vi "log analysis_gps.vi"() -> ()   [LabVIEW 2018] (continued)
283169.300,02000000,471d,15824;INS_ALIGNMENT_COMPLETE,INS_RTKFIXED,37.37108798474,126.72336907996,8.2218,22.3000,0.0121,0.0069,-0.0018,-0.383839466,-0.586517581,287.881593098,0.2239,0.1710,0.2714,0.0357,0.0355,0.0323,0.0788,0.0798,5.0127,0f000005,0*36e8c713\n\tsystem status\tnormal 2 28.000000 0 0\trobot status\t224.455343\t106.296732\t8.221800\t-0.383839\t-0.586518\t162.118407\t0.000000\t0.000000\n\t\n15:39:11.8\tlog_raw\tgps_raw\t#INSPVAXA,USB3,0,47.5,FINESTEERING,2107,283169.800,02000000,471d,15824;INS_ALIGNMENT_COMPLETE,INS_RTKFIXED,37.37108797168,126.72336907326,8.2216,22.3000,0.0108,0.0060,-0.0021,-0.382641749,-0.586060307,287.885088335,0.2239,0.1710,0.2714,0.0357,0.0355,0.0323,0.0788,0.0798,5.0127,0f000005,0*d441264a\n\tsystem status\tnormal 2 28.000000 0 0\trobot status\t224.454749\t106.295283\t8.221600\t-0.382642\t-0.586060\t162.114912\t0.000000\t0.000000\n\t\n15:39:12.3\tlog_raw\tgps_raw\t#INSPVAXA,USB3,0,49.5,FINESTEERING,2107,283170.300,02000000,471d,15824;INS_ALIGNMENT_COMPLETE,INS_RTKFIXED,37.37108796269,126.72336906818,8.2217,22.3000,0.0104,0.0055,-0.0014,-0.383475872,-0.583542182,287.889042259,0.2231,0.1689,0.2708,0.0348,0.0347,0.0316,0.0786,0.0797,5.0142,0f000005,0*32689bb7\n\tsystem status\tnormal 2 28.000000 0 0\trobot status\t224.454300\t106.294285\t8.221700\t-0.383476\t-0.583542\t162.110958\t0.000000\t0.000000\n\t\n15:39:12.8\tlog_raw\tgps_raw\t#INSPVAXA,USB3,0,49.5,FINESTEERING,2107,283170.800,02000000,471d,15824;INS_ALIGNMENT_COMPLETE,INS_RTKFIXED,37.37108796102,126.72336906813,8.2219,22.3000,0.0104,0.0056,-0.0013,-0.382678847,-0.583610963,287.888842190,0.2231,0.1689,0.2708,0.0348,0.0347,0.0316,0.0786,0.0797,5.0142,0f000005,0*5e85f202\n\tsystem status\tnormal 2 28.000000 0 0\trobot status\t224.454295\t106.294100\t8.221900\t-0.382679\t-0.583611\t162.111158\t0.000000\t0.000000\n\t\n15:39:13.3\tlog_raw\tgps_raw\t#INSPVAXA,USB3,0,48.5,FINESTEERING,2107,283171.300,02000000,471d,15824;INS_ALIGNMENT_COMPLETE,INS_RTKFIXED,37.37108796031,126.72336906830,8.2221,22.3000,0.0098,0.0065,-0.0020,-0.382671205,-0.583618137,287.888068003,0.2220,0.1670,0.2703,0.0345,0.0344,0.0314,0.0786,0.0797,5.0156,0f000005,0*d6c1e6dd\n\tsystem status\tnormal 2 28.000000 0 0\trobot status\t224.454310\t106.294021\t8.222100\t-0.382671\t-0.583618\t162.111932\t0.000000\t0.000000\n\t\n15:39:13.8\tlog_raw\tgps_raw\t#INSPVAXA,USB3,0,48.5,FINESTEERING,2107,283171.800,02000000,471d,15824;INS_ALIGNMENT_COMPLETE,INS_RTKFIXED,37.37108796545,126.72336907471,8.2220,22.3000,0.0105,0.0071,-0.0022,-0.380415359,-0.582586820,287.889750442,0.2220,0.1670,0.2703,0.0345,0.0344,0.0314,0.0786,0.0797,5.0156,0f000005,0*ca9dcfb0\n\tsystem status\tnormal 2 28.000000 0 0\trobot status\t224.454878\t106.294591\t8.222000\t-0.380415\t-0.582587\t162.110250\t0.000000\t0.000000\n\t\n15:39:14.3\tlog_raw\tgps_raw\t#INSPVAXA,USB3,0,50.0,FINESTEERING,2107,283172.300,02000000,471d,15824;INS_ALIGNMENT_COMPLETE,INS_RTKFIXED,37.37108796771,126.72336907645,8.2222,22.3000,0.0108,0.0068,-0.0016,-0.379539912,-0.580787545,287.890138856,0.2209,0.1652,0.2698,0.0344,0.0343,0.0313,0.0787,0.0798,5.0170,0f000005,0*259de970\n\tsystem status\tnormal 2 28.000000 0 0\trobot status\t224.455032\t106.294842\t8.222200\t-0.379540\t-0.580788\t162.109861\t0.000000\t0.000000\n\t\n15:39:14.8\tlog_raw\tgps_raw\t#INSPVAXA,USB3,0,50.0,FINESTEERING,2107,283172.800,02000000,471d,15824;INS_ALIGNMENT_COMPLETE,INS_RTKFIXED,37.37108797403,126.72336907678,8.2227,22.3000,0.0110,0.0071,-0.0014,-0.379066228,-0.579747038,287.892022667,0.2209,0.1652,0.2698,0.0344,0.0343,0.0313,0.0787,0.0798,5.0170,0f000005,0*0ecf865b\n\tsystem status\tnormal 2 28.000000 0 0\trobot status\t224.455061\t106.295543\t8.222700\t-0.379066\t-0.579747\t162.107977\t0.000000\t0.000000\n\t\n15:39:15.3\tlog_raw\tgps_raw\t#INSPVAXA,USB3,0,51.5,FINESTEERING,2107,283173.300,02000000,471d,15824;INS_ALIGNMENT_COMPLETE,INS_RTKFIXED,37.37108801209,126.72336910611,8.2226,22.3000,0.0136,0.0085,-0.0010,-0.377696334,-0.579038466,287.894073906,0.2209,0.1652,0.2698,0.0344,0.0343,0.0313,0.0787,0.0798,5.0170,0f000005,0*92cf69d3\n\tsystem status\tnormal 2 28.000000 0 0\trobot status\t224.457659\t106.299767\t8.222600\t-0.377696\t-0.579038\t162.105926\t0.000000\t0.000000\n\t\n15:39:15.8\tlog_raw\tgps_raw\t#INSPVAXA,USB3,0,51.5,FINESTEERING,2107,283173.800,02000000,471d,15824;INS_ALIGNMENT_COMPLETE,INS_RTKFIXED,37.37108808085,126.72336916289,8.2221,22.3000,0.0168,0.0112,-0.0008,-0.373536353,-0.577127426,287.890111312,0.2209,0.1652,0.2698,0.0344,0.0343,0.0313,0.0787,0.0798,5.0170,0f000005,0*81360348\n\tsystem status\tnormal 2 28.000000 0 0\trobot status\t224.462689\t106.307399\t8.222100\t-0.373536\t-0.577127\t162.109889\t0.000000\t0.000000\n\t\n15:39:16.3\tlog_raw\tgps_raw\t#DUALANTENNAHEADINGA,USB3,0,44.0,FINESTEERING,2107,283174.300,02000000,d426,15824;INSUFFICIENT_OBS,NONE,-1.000000000,0.000000000,0.000000000,0.0,0.000000000,0.000000000,\"631T\",17,4,4,3,04,00,20,03*70a0cfeb\n\tsystem status\tnormal 2 28.000000 0 0\trobot status\t224.463323\t106.308276\t8.222100\t-0.371384\t-0.577439\t162.106720\t0.000000\t0.000000\n\t\n15:39:16.8\tlog_raw\tgps_raw\t#DUALANTENNAHEADINGA,USB3,0,44.0,FINESTEERING,2107,283174.800,02000000,d426,15824;INSUFFICIENT_OBS,NONE,-1.000000000,0.000000000,0.000000000,0.0,0.000000000,0.000000000,\"631T\",15,4,4,3,04,00,20,03*9126eb2e\n\tsystem status\tnormal 2 28.000000 0 0\trobot status\t224.461054\t106.304461\t8.222600\t-0.374661\t-0.575974\t162.100760\t0.000000\t0.000000\n\t\n15:39:17.3\tlog_raw\tgps_raw\t#DUALANTENNAHEADINGA,USB3,0,49.0,FINESTEERING,2107,283175.300,02000000,d426,15824;INSUFFICIENT_OBS,NONE,-1.000000000,0.000000000,0.000000000,0.0,0.000000000,0.000000000,\"631T\",14,2,2,2,04,00,20,00*c59d9589\n\tsystem status\tnormal 2 28.000000 0 0\trobot status\t224.459353\t106.301886\t8.223100\t-0.378382\t-0.575410\t162.099451\t0.000000\t0.000000\n\t\n15:39:17.8\tlog_raw\tgps_raw\t#INSPVAXA,USB3,0,49.0,FINESTEERING,2107,283175.800,02000000,471d,15824;INS_ALIGNMENT_COMPLETE,INS_RTKFIXED,37.37108802047,126.72336911665,8.2237,22.3000,0.0129,0.0096,0.0019,-0.378938573,-0.573397489,287.902596878,0.2314,0.1754,0.2784,0.0357,0.0355,0.0323,0.0784,0.0795,5.0209,0f000005,0*65843865\n\tsystem status\tnormal 2 28.000000 0 0\trobot status\t224.458593\t106.300697\t8.223700\t-0.378939\t-0.573397\t162.097403\t0.000000\t0.000000\n\t\n15:39:18.3\tlog_raw\tgps_raw\t#INSPVAXA,USB3,0,50.0,FINESTEERING,2107,283176.300,02000000,471d,15824;INS_ALIGNMENT_COMPLETE,INS_RTKFIXED,37.37108801184,126.72336911067,8.2239,22.3000,0.0121,0.0095,0.0018,-0.379072967,-0.575586336,287.905355097,0.2295,0.1724,0.2772,0.0348,0.0346,0.0316,0.0783,0.0794,5.0222,0f000005,0*c18ce629\n\tsystem status\tnormal 2 28.000000 0 0\trobot status\t224.458063\t106.299740\t8.223900\t-0.379073\t-0.575586\t162.094645\t0.000000\t0.000000\n\t\n15:39:18.8\tlog_raw\tgps_raw\t#INSPVAXA,USB3,0,50.0,FINESTEERING,2107,283176.800,02000000,471d,15824;INS_ALIGNMENT_COMPLETE,INS_RTKFIXED,37.37108800756,126.72336910969,8.2238,22.3000,0.0114,0.0095,0.0012,-0.381926010,-0.578081656,287.907841439,0.2295,0.1724,0.2772,0.0348,0.0346,0.0316,0.0783,0.0794,5.0222,0f000005,0*ef194e5b\n\tsystem status\tnormal 2 28.000000 0 0\trobot status\t224.457976\t106.299265\t8.223800\t-0.381926\t-0.578082\t162.092159\t0.000000\t0.000000\n\t\n15:39:19.3\tlog_raw\tgps_raw\t#DUALANTENNAHEADINGA,USB3,0,49.0,FINESTEERING,2107,283177.300,02000000,d426,15824;INSUFFICIENT_OBS,NONE,-1.000000000,0.000000000,0.000000000,0.0,0.000000000,0.000000000,\"631T\",17,2,2,2,04,00,20,00*bd7b1a92\n\tsystem status\tnormal 2 28.000000 0 0\trobot status\t224.457745\t106.298989\t8.223800\t-0.383371\t-0.575370\t162.090491\t0.000000\t0.000000\n\t\n15:39:19.8\tlog_raw\tgps_raw\t#DUALANTENNAHEADINGA,USB3,0,49.0,FINESTEERING,2107,283177.800,02000000,d426,15824;INSUFFICIENT_OBS,NONE,-1.000000000,0.000000000,0.000000000,0.0,0.000000000,0.000000000,\"631T\",16,2,2,2,04,00,20,00*ffabb8fe\n\tsystem status\tnormal 2 28.000000 0 0\trobot status\t224.457983\t106.299228\t8.223800\t-0.382742\t-0.576805\t162.088762\t0.000000\t0.000000\n\t\n15:39:20.3\tlog_raw\tgps_raw\t#DUALANTENNAHEADINGA,USB3,0,48.5,FINESTEERING,2107,283178.300,02000000,d426,15824;INSUFFICIENT_OBS,NONE,-1.000000000,0.000000000,0.000000000,0.0,0.000000000,0.000000000,\"631T\",16,2,2,2,04,00,20,00*59fc98a6\n\tsystem status\tnormal 2 28.000000 0 0\trobot status\t224.458111\t106.299175\t8.223600\t-0.382875\t-0.576566\t162.089453\t0.000000\t0.000000\n\t\n15:39:20.8\tlog_raw\tgps_raw\t#INSPVAXA,USB3,0,48.5,FINESTEERING,2107,283178.800,02000000,471d,15824;INS_ALIGNMENT_COMPLETE,INS_RTKFIXED,37.37108800752,126.72336911614,8.2234,22.3000,0.0091,0.0098,0.0003,-0.383716997,-0.576517366,287.910600308,0.2256,0.1673,0.2752,0.0344,0.0343,0.0313,0.0786,0.0797,5.0251,0f000005,0*a6696e29\n\tsystem status\tnormal 2 28.000000 0 0\trobot status\t224.458548\t106.299260\t8.223400\t-0.383717\t-0.576517\t162.089400\t0.000000\t0.000000\n\t\n15:39:21.3\tlog_raw\tgps_raw\t#DUALANTENNAHEADINGA,USB3,0,49.5,FINESTEERING,2107,283179.300,02000000,d426,15824;INSUFFICIENT_OBS,NONE,-1.000000000,0.000000000,0.000000000,0.0,0.000000000,0.000000000,\"631T\",12,2,2,2,04,00,20,00*b9084739\n\tsystem status\tnormal 2 28.000000 0 0\trobot status\t224.458944\t106.298881\t8.223100\t-0.384356\t-0.576521\t162.085708\t0.000000\t0.000000\n\t\n15:39:21.8\tlog_raw\tgps_raw\t#INSPVAXA,USB3,0,49.5,FINESTEERING,2107,283179.800,02000000,471d,15824;INS_ALIGNMENT_COMPLETE,INS_RTKFIXED,37.37108800248,126.72336912231,8.2230,22.3000,0.0076,0.0089,-0.0004,-0.383606530,-0.576962847,287.915737403,0.2238,0.1653,0.2743,0.0344,0.0342,0.0313,0.0787,0.0798,5.0265,0f000005,0*ee90b331\n\tsystem status\tnormal 2 28.000000 0 0\trobot status\t224.459094\t106.298701\t8.223000\t-0.383607\t-0.576963\t162.084263\t0.000000\t0.000000\n\t\n15:39:22.3\tlog_raw\tgps_raw\t#INSPVAXA,USB3,0,48.5,FINESTEERING,2107,283180.300,02000000,471d,15824;INS_ALIGNMENT_COMPLETE,INS_RTKFIXED,37.37108799880,126.72336912044,8.2230,22.3000,0.0074,0.0084,-0.0003,-0.382763287,-0.577609398,287.917624770,0.2223,0.1637,0.2735,0.0344,0.0342,0.0312,0.0788,0.0799,5.0279,0f000005,0*b9fcfa2d\n\tsystem status\tnormal 2 28.000000 0 0\trobot status\t224.458929\t106.298292\t8.223000\t-0.382763\t-0.577609\t162.082375\t0.000000\t0.000000\n\t\n15:39:22.8\tlog_raw\tgps_raw\t#DUALANTENNAHEADINGA,USB3,0,48.5,FINESTEERING,2107,283180.800,02000000,d426,15824;INSUFFICIENT_OBS,NONE,-1.000000000,0.000000000,0.000000000,0.0,0.000000000,0.000000000,\"631T\",14,2,2,2,04,00,20,00*67370902\n\tsystem status\tnormal 2 28.000000 0 0\trobot status\t224.458826\t106.297985\t8.222800\t-0.381545\t-0.578104\t162.081748\t0.000000\t0.000000\n\t\n15:39:23.3\tlog_raw\tgps_raw\t#INSPVAXA,USB3,0,51.0,FINESTEERING,2107,283181.300,02000000,471d,15824;INS_ALIGNMENT_COMPLETE,INS_RTKFIXED,37.37108799142,126.72336911584,8.2227,22.3000,0.0062,0.0073,-0.0012,-0.379070208,-0.579479951,287.919184058,0.2209,0.1624,0.2727,0.0344,0.0342,0.0312,0.0789,0.0800,5.0294,0f000005,0*ff5c7a42\n\tsystem status\tnormal 2 28.000000 0 0\trobot status\t224.458521\t106.297473\t8.222700\t-0.379070\t-0.579480\t162.080816\t0.000000\t0.000000\n\t\n15:39:23.8\tlog_raw\tgps_raw\t#INSPVAXA,USB3,0,51.0,FINESTEERING,2107,283181.800,02000000,471d,15824;INS_ALIGNMENT_COMPLETE,INS_RTKFIXED,37.37108798938,126.72336911647,8.2229,22.3000,0.0064,0.0075,-0.0013,-0.378914786,-0.582250994,287.920027881,0.2209,0.1624,0.2727,0.0344,0.0342,0.0312,0.0789,0.0800,5.0294,0f000005,0*210c1369\n\tsystem status\tnormal 2 28.000000 0 0\trobot status\t224.458577\t106.297247\t8.222900\t-0.378915\t-0.582251\t162.079972\t0.000000\t0.000000\n\t\n15:39:24.3\tlog_raw\tgps_raw\t#INSPVAXA,USB3,0,50.5,FINESTEERING,2107,283182.300,02000000,471d,15824;INS_ALIGNMENT_COMPLETE,INS_RTKFIXED,37.37108798784,126.72336911574,8.2231,22.3000,0.0069,0.0073,-0.0014,-0.376950030,-0.581137760,287.919196566,0.2197,0.1614,0.2720,0.0344,0.0342,0.0312,0.0790,0.0800,5.0308,0f000005,0*5d6efddc\n\tsystem status\tnormal 2 28.000000 0 0\trobot status\t224.458512\t106.297076\t8.223100\t-0.376950\t-0.581138\t162.080803\t0.000000\t0.000000\n\t\n15:39:24.8\tlog_raw\tgps_raw\t#INSPVAXA,USB3,0,50.5,FINESTEERING,2107,283182.800,02000000,471d,15824;INS_ALIGNMENT_COMPLETE,INS_RTKFIXED,37.37108799276,126.72336911883,8.2233,22.3000,0.0080,0.0075,-0.0014,-0.377644437,-0.581747143,287.919278227,0.2197,0.1614,0.2720,0.0344,0.0342,0.0312,0.0790,0.0800,5.0308,0f000005,0*2c1378c7\n\tsystem status\tnormal 2 28.000000 0 0\trobot status\t224.458786\t106.297622\t8.223300\t-0.377644\t-0.581747\t162.080722\t0.000000\t0.000000\n\t\n15:39:25.3\tlog_raw\tgps_raw\t#INSPVAXA,USB3,0,50.0,FINESTEERING,2107,283183.300,02000000,471d,15824;INS_ALIGNMENT_COMPLETE,INS_RTKFIXED,37.37108799440,126.72336911810,8.2235,22.3000,0.0083,0.0077,-0.0003,-0.377907999,-0.580976107,287.918524275,0.2187,0.1605,0.2713,0.0344,0.0342,0.0312,0.0791,0.0801,5.0323,0f000005,0*3971cbaa\n\tsystem status\tnormal 2 28.000000 0 0\trobot status\t224.458721\t106.297804\t8.223500\t-0.377908\t-0.580976\t162.081476\t0.000000\t0.000000\n\t\n15:39:25.8\tlog_raw\tgps_raw\t#DUALANTENNAHEADINGA,USB3,0,50.0,FINESTEERING,2107,283183.800,02000000,d426,15824;INSUFFICIENT_OBS,NONE,-1.000000000,0.000000000,0.000000000,0.0,0.000000000,0.000000000,\"631T\",15,2,2,2,04,00,20,00*16dcf878\n\tsystem status\tnormal 2 28.000000 0 0\trobot status\t224.458618\t106.297862\t8.223900\t-0.378860\t-0.580270\t162.080455\t0.000000\t0.000000\n\t\n15:39:26.3\tlog_raw\tgps_raw\t#INSPVAXA,USB3,0,49.5,FINESTEERING,2107,283184.300,02000000,471d,15824;INS_ALIGNMENT_COMPLETE,INS_RTKFIXED,37.37108799290,126.72336911350,8.2241,22.3000,0.0072,0.0062,0.0001,-0.380085189,-0.579242316,287.919684164,0.2178,0.1599,0.2707,0.0344,0.0343,0.0312,0.0792,0.0801,5.0339,0f000005,0*bc5fd1df\n\tsystem status\tnormal 2 28.000000 0 0\trobot status\t224.458314\t106.297638\t8.224100\t-0.380085\t-0.579242\t162.080316\t0.000000\t0.000000\n\t\n15:39:26.8\tlog_raw\tgps_raw\t#DUALANTENNAHEADINGA,USB3,0,49.5,FINESTEERING,2107,283184.800,02000000,d426,15824;INSUFFICIENT_OBS,NONE,-1.000000000,0.000000000,0.000000000,0.0,0.000000000,0.000000000,\"631T\",15,2,2,2,04,00,20,00*b8804adb\n\tsystem status\tnormal 2 28.000000 0 0\trobot status\t224.458148\t106.297609\t8.224200\t-0.378372\t-0.579532\t162.077791\t0.000000\t0.000000\n\t\n15:39:27.3\tlog_raw\tgps_raw\t#INSPVAXA,USB3,0,51.0,FINESTEERING,2107,283185.300,02000000,471d,15824;INS_ALIGNMENT_COMPLETE,INS_RTKFIXED,37.37108798957,126.72336910890,8.2243,22.3000,0.0072,0.0065,0.0004,-0.376376594,-0.581358564,287.922376317,0.2170,0.1594,0.2701,0.0344,0.0343,0.0312,0.0792,0.0802,5.0354,0f000005,0*e79d958c\n\tsystem status\tnormal 2 28.000000 0 0\trobot status\t224.457906\t106.297268\t8.224300\t-0.376377\t-0.581359\t162.077624\t0.000000\t0.000000\n\t\n15:39:27.8\tlog_raw\tgps_raw\t#DUALANTENNAHEADINGA,USB3,0,51.0,FINESTEERING,2107,283185.800,02000000,d426,15824;INSUFFICIENT_OBS,NONE,-1.000000000,0.000000000,0.000000000,0.0,0.000000000,0.000000000,\"631T\",15,2,2,2,04,00,20,00*c539324b\n\tsystem status\tnormal 2 28.000000 0 0\trobot status\t224.457938\t106.297132\t8.224300\t-0.376262\t-0.582809\t162.075708\t0.000000\t0.000000\n\t\n15:39:28.3\tlog_raw\tgps_raw\t#INSPVAXA,USB3,0,49.5,FINESTEERING,2107,283186.300,02000000,471d,15824;INS_ALIGNMENT_COMPLETE,INS_RTKFIXED,37.37108798620,126.72336910856,8.2243,22.3000,0.0071,0.0073,-0.0002,-0.377506910,-0.583623217,287.927831882,0.2163,0.1590,0.2696,0.0344,0.0343,0.0312,0.0792,0.0802,5.0369,0f000005,0*21523d82\n\tsystem status\tnormal 2 28.000000 0 0\trobot status\t224.457876\t106.296894\t8.224300\t-0.377507\t-0.583623\t162.072168\t0.000000\t0.000000\n\t\n15:39:28.8\tlog_raw\tgps_raw\t#DUALANTENNAHEADINGA,USB3,0,49.5,FINESTEERING,2107,283186.800,02000000,d426,15824;INSUFFICIENT_OBS,NONE,-1.000000000,0.000000000,0.000000000,0.0,0.000000000,0.000000000,\"631T\",14,4,4,3,04,00,20,03*758328f4\n\tsystem status\tnormal 2 28.000000 0 0\trobot status\t224.458116\t106.296703\t8.224100\t-0.378999\t-0.585177\t162.072040\t0.000000\t0.000000\n\t\n15:39:29.3\tlog_raw\tgps_raw\t#INSPVAXA,USB3,0,46.0,FINESTEERING,2107,283187.300,02000000,471d,15824;INS_ALIGNMENT_COMPLETE,INS_RTKFIXED,37.37108798055,126.72336910974,8.2240,22.3000,0.0067,0.0070,0.0001,-0.381669916,-0.586056120,287.928395893,0.2158,0.1586,0.2691,0.0344,0.0343,0.0312,0.0793,0.0802,5.0384,0f000005,0*68985769\n\tsystem status\tnormal 2 28.000000 0 0\trobot status\t224.457981\t106.296267\t8.224000\t-0.381670\t-0.586056\t162.071604\t0.000000\t0.000000\n\t\n15:39:29.8\tlog_raw\tgps_raw\t#INSPVAXA,USB3,0,46.0,FINESTEERING,2107,283187.800,02000000,471d,15824;INS_ALIGNMENT_COMPLETE,INS_RTKFIXED,37.37108797480,126.72336910787,8.2241,22.3000,0.0056,0.0073,-0.0002,-0.384514938,-0.587125643,287.930034096,0.2158,0.1586,0.2691,0.0344,0.0343,0.0312,0.0793,0.0802,5.0384,0f000005,0*a7c7a978\n\tsystem status\tnormal 2 28.000000 0 0\trobot status\t224.457815\t106.295629\t8.224100\t-0.384515\t-0.587126\t162.069966\t0.000000\t0.000000\n\t\n15:39:30.3\tlog_raw\tgps_raw\t#DUALANTENNAHEADINGA,USB3,0,50.5,FINESTEERING,2107,283188.300,02000000,d426,15824;INSUFFICIENT_OBS,NONE,-1.000000000,0.000000000,0.000000000,0.0,0.000000000,0.000000000,\"631T\",15,2,2,2,04,00,20,00*b8de1ba1\n\tsystem status\tnormal 2 28.000000 0 0\trobot status\t224.457651\t106.294918\t8.224000\t-0.384438\t-0.586820\t162.068385\t0.000000\t0.000000\n\t\n15:39:30.8\tlog_raw\tgps_raw\t#INSPVAXA,USB3,0,50.5,FINESTEERING,2107,283188.800,02000000,471d,15824;INS_ALIGNMENT_COMPLETE,INS_RTKFIXED,37.37108796465,126.72336910438,8.2240,22.3000,0.0044,0.0069,-0.0006,-0.384553588,-0.585982152,287.932075352,0.2153,0.1584,0.2687,0.0344,0.0343,0.0312,0.0793,0.0802,5.0398,0f000005,0*584615a0\n\tsystem status\tnormal 2 28.000000 0 0\trobot status\t224.457506\t106.294502\t8.224000\t-0.384554\t-0.585982\t162.067925\t0.000000\t0.000000\n\t\n15:39:31.3\tlog_raw\tgps_raw\t#DUALANTENNAHEADINGA,USB3,0,50.0,FINESTEERING,2107,283189.300,02008000,d426,15824;SOL_COMPUTED,L1_FLOAT,-1.000000000,22.943321228,-27.912841797,0.0,360.000000000,180.000000000,\"631T\",17,5,5,3,04,00,20,03*61e408ae\n\tsystem status\tnormal 2 28.000000 0 0\trobot status\t224.457320\t106.293974\t8.224100\t-0.385036\t-0.586456\t162.066713\t0.000000\t0.000000\n\t\n15:39:31.8\tlog_raw\tgps_raw\t#INSPVAXA,USB3,0,50.0,FINESTEERING,2107,283189.800,02008000,471d,15824;INS_ALIGNMENT_COMPLETE,INS_RTKFIXED,37.37108795686,126.72336910595,8.2245,22.3000,0.0035,0.0080,-0.0003,-0.386062307,-0.585594940,287.936481773,0.2149,0.1582,0.2683,0.0344,0.0343,0.0312,0.0793,0.0802,5.0412,0f000005,0*927e0823\n\tsystem status\tnormal 2 28.000000 0 0\trobot status\t224.457645\t106.293638\t8.224500\t-0.386062\t-0.585595\t162.063518\t0.000000\t0.000000\n\t\n15:39:32.3\tlog_raw\tgps_raw\t#DUALANTENNAHEADINGA,USB3,0,46.5,FINESTEERING,2107,283190.300,02008000,d426,15824;SOL_COMPUTED,L1_FLOAT,-1.000000000,295.270263672,43.260082245,0.0,360.000000000,180.000000000,\"631T\",14,5,5,3,04,00,20,03*6a966b3f\n\tsystem status\tnormal 2 28.000000 0 0\trobot status\t224.457739\t106.293105\t8.224900\t-0.386580\t-0.587024\t162.064370\t0.000000\t0.000000\n\t\n15:39:32.8\tlog_raw\tgps_raw\t#DUALANTENNAHEADINGA,USB3,0,46.5,FINESTEERING,2107,283190.800,02008000,d426,15824;SOL_COMPUTED,L1_FLOAT,-1.000000000,350.638061523,5.315610409,0.0,360.000000000,180.000000000,\"631T\",13,5,5,3,04,00,20,03*8fee928e\n\tsystem status\tnormal 2 28.000000 0 0\trobot status\t224.457246\t106.293053\t8.225100\t-0.389434\t-0.587141\t162.064854\t0.000000\t0.000000\n\t\n15:39:33.3\tlog_raw\tgps_raw\t#DUALANTENNAHEADINGA,USB3,0,51.0,FINESTEERING,2107,283191.300,02008000,d426,15824;SOL_COMPUTED,L1_FLOAT,-1.000000000,12.310025215,-18.113586426,0.0,360.000000000,180.000000000,\"631T\",14,5,5,3,04,00,20,03*cb2a916c\n\tsystem status\tnormal 2 28.000000 0 0\trobot status\t224.457686\t106.293094\t8.225300\t-0.387481\t-0.588588\t162.062776\t0.000000\t0.000000\n\t\n15:39:33.8\tlog_raw\tgps_raw\t#DUALANTENNAHEADINGA,USB3,0,51.0,FINESTEERING,2107,283191.800,02008000,d426,15824;SOL_COMPUTED,L1_FLOAT,-1.000000000,35.111301422,-35.377624512,0.0,101.695205688,180.000000000,\"631T\",14,5,5,3,04,00,20,03*191bd153\n\tsystem status\tnormal 2 28.000000 0 0\trobot status\t224.458001\t106.293764\t8.225500\t-0.387985\t-0.588111\t162.062664\t0.000000\t0.000000\n\t\n15:39:34.3\tlog_raw\tgps_raw\t#INSPVAXA,USB3,0,48.0,FINESTEERING,2107,283192.300,02008000,471d,15824;INS_ALIGNMENT_COMPLETE,INS_RTKFIXED,37.37108795667,126.72336911311,8.2256,22.3000,0.0046,0.0093,0.0005,-0.387858319,-0.587901427,287.938370105,0.2139,0.1579,0.2673,0.0344,0.0343,0.0312,0.0793,0.0802,5.0456,0f000005,0*318753ed\n\tsystem status\tnormal 2 28.000000 0 0\trobot status\t224.458279\t106.293617\t8.225600\t-0.387858\t-0.587901\t162.061630\t0.000000\t0.000000\n\t\n15:39:34.8\tlog_raw\tgps_raw\t#DUALANTENNAHEADINGA,USB3,0,48.0,FINESTEERING,2107,283192.800,02008000,d426,15824;SOL_COMPUTED,L1_FLOAT,-1.000000000,28.920713425,-31.830932617,0.0,228.720611572,180.000000000,\"631T\",14,5,5,3,04,00,20,03*dfadfb53\n\tsystem status\tnormal 2 28.000000 0 0\trobot status\t224.459151\t106.293046\t8.225300\t-0.387927\t-0.587382\t162.060913\t0.000000\t0.000000\n\t\n15:39:35.3\tlog_raw\tgps_raw\t#DUALANTENNAHEADINGA,USB3,0,52.5,FINESTEERING,2107,283193.300,02008000,d426,15824;SOL_COMPUTED,L1_FLOAT,-1.000000000,22.577627182,-27.194854736,0.0,360.000000000,180.000000000,\"631T\",14,5,5,3,04,00,20,03*2b92c623\n\tsystem status\tnormal 2 28.000000 0 0\trobot status\t224.459506\t106.292527\t8.224900\t-0.389172\t-0.588703\t162.060098\t0.000000\t0.000000\n\t\n15:39:35.8\tlog_raw\tgps_raw\t#INSPVAXA,USB3,0,52.5,FINESTEERING,2107,283193.800,02008000,471d,15824;INS_ALIGNMENT_COMPLETE,INS_RTKFIXED,37.37108794696,126.72336913145,8.2245,22.3000,0.0046,0.0096,-0.0011,-0.386759073,-0.585024800,287.941284128,0.2137,0.1578,0.2670,0.0344,0.0343,0.0312,0.0793,0.0802,5.0469,0f000005,0*303171d6\n\tsystem status\tnormal 2 28.000000 0 0\trobot status\t224.459904\t106.292539\t8.224500\t-0.386759\t-0.585025\t162.058716\t0.000000\t0.000000\n\t\n15:39:36.3\tlog_raw\tgps_raw\t#INSPVAXA,USB3,0,47.5,FINESTEERING,2107,283194.300,02008000,471d,15824;INS_ALIGNMENT_COMPLETE,INS_RTKFIXED,37.37108794768,126.72336913167,8.2241,22.3000,0.0062,0.0083,-0.0013,-0.387313384,-0.586457322,287.941677020,0.2135,0.1577,0.2667,0.0344,0.0343,0.0312,0.0793,0.0802,5.0484,0f000005,0*fb34fba9\n\tsystem status\tnormal 2 28.000000 0 0\trobot status\t224.459923\t106.292619\t8.224100\t-0.387313\t-0.586457\t162.058323\t0.000000\t0.000000\n\t\n15:39:36.8\tlog_raw\tgps_raw\t#DUALANTENNAHEADINGA,USB3,0,47.5,FINESTEERING,2107,283194.800,02008000,d426,15824;SOL_COMPUTED,L1_FLOAT,-1.000000000,15.914994240,-22.873901367,0.0,360.000000000,180.000000000,\"631T\",14,5,5,3,04,00,20,03*a57ffdb4\n\tsystem status\tnormal 2 28.000000 0 0\trobot status\t224.459643\t106.293299\t8.224000\t-0.384843\t-0.589820\t162.060407\t0.000000\t0.000000\n\t\n15:39:37.3\tlog_raw\tgps_raw\t#DUALANTENNAHEADINGA,USB3,0,50.5,FINESTEERING,2107,283195.300,02008000,d426,15824;INSUFFICIENT_OBS,NONE,-1.000000000,0.000000000,0.000000000,0.0,0.000000000,0.000000000,\"631T\",14,4,4,4,04,00,20,20*483b483f\n\tsystem status\tnormal 2 28.000000 0 0\trobot status\t224.459443\t106.293499\t8.224100\t-0.384960\t-0.589704\t162.059334\t0.000000\t0.000000\n\t\n15:39:37.8\tlog_raw\tgps_raw\t#DUALANTENNAHEADINGA,USB3,0,50.5,FINESTEERING,2107,283195.800,02008000,d426,15824;INSUFFICIENT_OBS,NONE,-1.000000000,0.000000000,0.000000000,0.0,0.000000000,0.000000000,\"631T\",16,4,4,4,04,00,20,20*a9bd6cfa\n\tsystem status\tnormal 2 28.000000 0 0\trobot status\t224.459364\t106.293637\t8.224200\t-0.385177\t-0.590148\t162.058176\t0.000000\t0.000000\n\t\n15:39:38.3\tlog_raw\tgps_raw\t#DUALANTENNAHEADINGA,USB3,0,48.5,FINESTEERING,2107,283196.300,02008000,d426,15824;INSUFFICIENT_OBS,NONE,-1.000000000,0.000000000,0.000000000,0.0,0.000000000,0.000000000,\"631T\",16,4,4,4,04,00,20,20*cffcd920\n\tsystem status\tnormal 2 28.000000 0 0\trobot status\t224.459020\t106.293658\t8.224500\t-0.386184\t-0.590996\t162.056646\t0.000000\t0.000000\n\t\n15:39:38.8\tlog_raw\tgps_raw\t#DUALANTENNAHEADINGA,USB3,0,48.5,FINESTEERING,2107,283196.800,02008000,d426,15824;INSUFFICIENT_OBS,NONE,-1.000000000,0.000000000,0.000000000,0.0,0.000000000,0.000000000,\"631T\",16,4,4,4,04,00,20,20*5acefb14\n\tsystem status\tnormal 2 28.000000 0 0\trobot status\t224.458755\t106.294009\t8.224900\t-0.389629\t-0.592443\t162.055876\t0.000000\t0.000000\n\t\n15:39:39.3\tlog_raw\tgps_raw\t#DUALANTENNAHEADINGA,USB3,0,49.0,FINESTEERING,2107,283197.300,02008000,d426,15824;INSUFFICIENT_OBS,NONE,-1.000000000,0.000000000,0.000000000,0.0,0.000000000,0.000000000,\"631T\",16,4,4,4,04,00,20,20*931aed91\n\tsystem status\tnormal 2 28.000000 0 0\trobot status\t224.458397\t106.293948\t8.225000\t-0.391871\t-0.592747\t162.056664\t0.000000\t0.000000\n\t\n15:39:39.8\tlog_raw\tgps_raw\t#DUALANTENNAHEADINGA,USB3,0,49.0,FINESTEERING,2107,283197.800,02008000,d426,15824;INSUFFICIENT_OBS,NONE,-1.000000000,0.000000000,0.000000000,0.0,0.000000000,0.000000000,\"631T\",16,4,4,4,04,00,20,20*0628cfa5\n\tsystem status\tnormal 2 28.000000 0 0\trobot status\t224.458046\t106.294286\t8.224600\t-0.392125\t-0.594160\t162.060691\t0.000000\t0.000000\n\t\n15:39:40.3\tlog_raw\tgps_raw\t#DUALANTENNAHEADINGA,USB3,0,48.5,FINESTEERING,2107,283198.300,02000000,d426,15824;SOL_COMPUTED,L1_FLOAT,-1.000000000,255.227523804,12.823373795,0.0,360.000000000,180.000000000,\"631T\",14,5,5,4,04,00,20,03*2801eac2\n\tsystem status\tnormal 2 28.000000 0 0\trobot status\t224.457685\t106.294450\t8.224500\t-0.392945\t-0.593265\t162.061074\t0.000000\t0.000000\n\t\n15:39:40.8\tlog_raw\tgps_raw\t#DUALANTENNAHEADINGA,USB3,0,48.5,FINESTEERING,2107,283198.800,02000000,d426,15824;SOL_COMPUTED,L1_FLOAT,-1.000000000,26.448829651,-49.172851563,0.0,283.970214844,136.538162231,\"631T\",14,5,5,4,04,00,20,03*767a920f\n\tsystem status\tnormal 2 28.000000 0 0\trobot status\t224.457330\t106.294836\t8.224600\t-0.394967\t-0.594915\t162.062724\t0.000000\t0.000000\n\t\n15:39:41.3\tlog_raw\tgps_raw\t#DUALANTENNAHEADINGA,USB3,0,48.5,FINESTEERING,2107,283199.300,02000000,d426,15824;INSUFFICIENT_OBS,NONE,-1.000000000,0.000000000,0.000000000,0.0,0.000000000,0.000000000,\"631T\",15,4,4,3,04,00,20,03*ae2edc4c\n\tsystem status\tnormal 2 28.000000 0 0\trobot status\t224.457034\t106.295038\t8.224600\t-0.394529\t-0.596676\t162.064286\t0.000000\t0.000000\n\t\n15:39:41.8\tlog_raw\tgps_raw\t#DUALANTENNAHEADINGA,USB3,0,48.5,FINESTEERING,2107,283199.800,02000000,d426,15824;INSUFFICIENT_OBS,NONE,-1.000000000,0.000000000,0.000000000,0.0,0.000000000,0.000000000,\"631T\",16,4,4,3,04,00,20,03*984a78d1\n\tsystem status\tnormal 2 28.000000 0 0\trobot status\t224.456962\t106.295329\t8.224600\t-0.395652\t-0.597678\t162.065364\t0.000000\t0.000000\n\t\n15:39:42.3\tlog_raw\tgps_raw\t#DUALANTENNAHEADINGA,USB3,0,47.0,FINESTEERING,2107,283200.300,02000000,d426,15824;INSUFFICIENT_OBS,NONE,-1.000000000,0.000000000,0.000000000,0.0,0.000000000,0.000000000,\"631T\",14,4,4,3,04,00,20,03*7a2c4abd\n\tsystem status\tnormal 2 28.000000 0 0\trobot status\t224.456698\t106.295245\t8.224600\t-0.398740\t-0.598802\t162.067151\t0.000000\t0.000000\n\t\n15:39:42.8\tlog_raw\tgps_raw\t#DUALANTENNAHEADINGA,USB3,0,47.0,FINESTEERING,2107,283200.800,02000000,d426,15824;INSUFFICIENT_OBS,NONE,-1.000000000,0.000000000,0.000000000,0.0,0.000000000,0.000000000,\"631T\",14,4,4,3,04,00,20,03*ef1e6889\n\tsystem status\tnormal 2 28.000000 0 0\trobot status\t224.456226\t106.295008\t8.224900\t-0.398532\t-0.599340\t162.068089\t0.000000\t0.000000\n\t\n15:39:43.3\tlog_raw\tgps_raw\t#DUALANTENNAHEADINGA,USB3,0,50.0,FINESTEERING,2107,283201.300,02000000,d426,15824;INSUFFICIENT_OBS,NONE,-1.000000000,0.000000000,0.000000000,0.0,0.000000000,0.000000000,\"631T\",15,2,2,2,04,00,20,00*363721e3\n\tsystem status\tnormal 2 28.000000 0 0\trobot status\t224.455700\t106.294825\t8.225000\t-0.401108\t-0.599995\t162.069768\t0.000000\t0.000000\n\t\n15:39:43.8\tlog_raw\tgps_raw\t#DUALANTENNAHEADINGA,USB3,0,50.0,FINESTEERING,2107,283201.800,02000000,d426,15824;INSUFFICIENT_OBS,NONE,-1.000000000,0.000000000,0.000000000,0.0,0.000000000,0.000000000,\"631T\",16,2,2,2,04,00,20,00*0053857e\n\tsystem status\tnormal 2 28.000000 0 0\trobot status\t224.455351\t106.294543\t8.224600\t-0.401356\t-0.598855\t162.072467\t0.000000\t0.000000\n\t\n15:39:44.3\tlog_raw\tgps_raw\t#DUALANTENNAHEADINGA,USB3,0,47.5,FINESTEERING,2107,283202.300,02000000,d426,15824;INSUFFICIENT_OBS,NONE,-1.000000000,0.000000000,0.000000000,0.0,0.000000000,0.000000000,\"631T\",15,2,2,2,04,00,20,00*e255ce5e\n\tsystem status\tnormal 2 28.000000 0 0\trobot status\t224.454992\t106.294104\t8.224100\t-0.403575\t-0.599361\t162.074506\t0.000000\t0.000000\n\t\n15:39:44.8\tlog_raw\tgps_raw\t#DUALANTENNAHEADINGA,USB3,0,47.5,FINESTEERING,2107,283202.800,02000000,d426,15824;INSUFFICIENT_OBS,NONE,-1.000000000,0.000000000,0.000000000,0.0,0.000000000,0.000000000,\"631T\",14,2,2,2,04,00,20,00*a0856c32\n\tsystem status\tnormal 2 28.000000 0 0\trobot status\t224.454715\t106.293983\t8.223600\t-0.404007\t-0.601663\t162.075621\t0.000000\t0.000000\n\t\n15:39:45.3\tlog_raw\tgps_raw\t#DUALANTENNAHEADINGA,USB3,0,48.5,FINESTEERING,2107,283203.300,02000000,d426,15824;INSUFFICIENT_OBS,NONE,-1.000000000,0.000000000,0.000000000,0.0,0.000000000,0.000000000,\"631T\",16,2,2,2,04,00,20,00*5eb0d2b1\n\tsystem status\tnormal 2 28.000000 0 0\trobot status\t224.454377\t106.293667\t8.223400\t-0.404109\t-0.599704\t162.076848\t0.000000\t0.000000\n\t\n15:39:45.8\tlog_raw\tgps_raw\t#DUALANTENNAHEADINGA,USB3,0,48.5,FINESTEERING,2107,283203.800,02000000,d426,15824;INSUFFICIENT_OBS,NONE,-1.000000000,0.000000000,0.000000000,0.0,0.000000000,0.000000000,\"631T\",16,2,2,2,04,00,20,00*cb82f085\n\tsystem status\tnormal 2 28.000000 0 0\trobot status\t224.453619\t106.293492\t8.223600\t-0.404832\t-0.598865\t162.078323\t0.000000\t0.000000\n\t\n15:39:46.3\tlog_raw\tgps_raw\t#DUALANTENNAHEADINGA,USB3,0,47.5,FINESTEERING,2107,283204.300,02000000,d426,15824;INSUFFICIENT_OBS,NONE,-1.000000000,0.000000000,0.000000000,0.0,0.000000000,0.000000000,\"631T\",18,2,2,2,04,00,20,00*62df42f6\n\tsystem status\tnormal 2 28.000000 0 0\trobot status\t224.452894\t106.293374\t8.223500\t-0.403683\t-0.598053\t162.076213\t0.000000\t0.000000\n\t\n15:39:46.8\tlog_raw\tgps_raw\t#DUALANTENNAHEADINGA,USB3,0,47.5,FINESTEERING,2107,283204.800,02000000,d426,15824;INSUFFICIENT_OBS,NONE,-1.000000000,0.000000000,0.000000000,0.0,0.000000000,0.000000000,\"631T\",17,2,2,2,04,00,20,00*b472f60c\n\tsystem status\tnormal 2 28.000000 0 0\trobot status\t224.452248\t106.293540\t8.223400\t-0.405042\t-0.596600\t162.074723\t0.000000\t0.000000\n\t\n15:39:47.3\tlog_raw\tgps_raw\t#DUALANTENNAHEADINGA,USB3,0,46.5,FINESTEERING,2107,283205.300,02000000,d426,15824;INSUFFICIENT_OBS,NONE,-1.000000000,0.000000000,0.000000000,0.0,0.000000000,0.000000000,\"631T\",15,2,2,2,04,00,20,00*5c6800b4\n\tsystem status\tnormal 2 28.000000 0 0\trobot status\t224.451802\t106.293289\t8.223100\t-0.406507\t-0.596259\t162.076191\t0.000000\t0.000000\n\t\n15:39:47.8\tlog_raw\tgps_raw\t#DUALANTENNAHEADINGA,USB3,0,46.5,FINESTEERING,2107,283205.800,02000000,d426,15824;INSUFFICIENT_OBS,NONE,-1.000000000,0.000000000,0.000000000,0.0,0.000000000,0.000000000,\"631T\",15,2,2,2,04,00,20,00*c95a2280\n\tsystem status\tnormal 2 28.000000 0 0\trobot status\t224.451645\t106.292751\t8.222600\t-0.408764\t-0.594850\t162.076971\t0.000000\t0.000000\n\t\n15:39:48.3\tlog_raw\tgps_raw\t#DUALANTENNAHEADINGA,USB3,0,49.0,FINESTEERING,2107,283206.300,02000000,d426,15824;INSUFFICIENT_OBS,NONE,-1.000000000,0.000000000,0.000000000,0.0,0.000000000,0.000000000,\"631T\",14,2,2,2,04,00,20,00*1af3f5d4\n\tsystem status\tnormal 2 28.000000 0 0\trobot status\t224.451356\t106.292200\t8.222500\t-0.408574\t-0.594064\t162.076610\t0.000000\t0.000000\n\t\n15:39:48.8\tlog_raw\tgps_raw\t#DUALANTENNAHEADINGA,USB3,0,49.0,FINESTEERING,2107,283206.800,02000000,d426,15824;INSUFFICIENT_OBS,NONE,-1.000000000,0.000000000,0.000000000,0.0,0.000000000,0.000000000,\"631T\",13,2,2,2,04,00,20,00*c5ff5cab\n\tsystem status\tnormal 2 28.000000 0 0\trobot status\t224.450977\t106.291899\t8.222500\t-0.406848\t-0.593356\t162.075811\t0.000000\t0.000000\n\t\n15:39:49.3\tlog_raw\tgps_raw\t#DUALANTENNAHEADINGA,USB3,0,49.5,FINESTEERING,2107,283207.300,02000000,d426,15824;INSUFFICIENT_OBS,NONE,-1.000000000,0.000000000,0.000000000,0.0,0.000000000,0.000000000,\"631T\",12,2,2,2,04,00,20,00*bf8d1cd2\n\tsystem status\tnormal 2 28.000000 0 0\trobot status\t224.450700\t106.291461\t8.222600\t-0.404874\t-0.592411\t162.074385\t0.000000\t0.000000\n\t\n15:39:49.8\tlog_raw\tgps_raw\t#DUALANTENNAHEADINGA,USB3,0,49.5,FINESTEERING,2107,283207.800,02000000,d426,15824;INSUFFICIENT_OBS,NONE,-1.000000000,0.000000000,0.000000000,0.0,0.000000000,0.000000000,\"631T\",12,2,2,2,04,00,20,00*2abf3ee6\n\tsystem status\tnormal 2 28.000000 0 0\trobot status\t224.450798\t106.291298\t8.222800\t-0.401983\t-0.591821\t162.074988\t0.000000\t0.000000\n\t\n15:39:50.3\tlog_raw\tgps_raw\t#DUALANTENNAHEADINGA,USB3,0,47.0,FINESTEERING,2107,283208.300,02000000,d426,15824;INSUFFICIENT_OBS,NONE,-1.000000000,0.000000000,0.000000000,0.0,0.000000000,0.000000000,\"631T\",14,4,4,3,04,00,20,03*a20e60f7\n\tsystem status\tnormal 2 28.000000 0 0\trobot status\t224.450864\t106.291238\t8.222900\t-0.399973\t-0.589450\t162.075342\t0.000000\t0.000000\n\t\n15:39:50.8\tlog_raw\tgps_raw\t#DUALANTENNAHEADINGA,USB3,0,47.0,FINESTEERING,2107,283208.800,02000000,d426,15824;INSUFFICIENT_OBS,NONE,-1.000000000,0.000000000,0.000000000,0.0,0.000000000,0.000000000,\"631T\",15,4,4,3,04,00,20,03*e0dec29b\n\tsystem status\tnormal 2 28.000000 0 0\trobot status\t224.450757\t106.291653\t8.222900\t-0.399417\t-0.590766\t162.075487\t0.000000\t0.000000\n\t\n15:39:51.3\tlog_raw\tgps_raw\t#DUALANTENNAHEADINGA,USB3,0,47.5,FINESTEERING,2107,283209.300,02000000,d426,15824;INSUFFICIENT_OBS,NONE,-1.000000000,0.000000000,0.000000000,0.0,0.000000000,0.000000000,\"631T\",14,4,4,3,04,00,20,03*9aac82e2\n\tsystem status\tnormal 2 28.000000 0 0\trobot status\t224.450659\t106.291752\t8.222900\t-0.400258\t-0.591304\t162.075615\t0.000000\t0.000000\n\t\n15:39:51.8\tlog_raw\tgps_raw\t#INSPVAXA,USB3,0,47.5,FINESTEERING,2107,283209.850,02000000,471d,15824;INS_ALIGNMENT_COMPLETE,INS_RTKFIXED,37.37108793670,126.72336902912,8.2230,22.3000,0.0057,0.0015,0.0021,-0.400587739,-0.588760253,287.923723239,0.2124,0.1575,0.2644,0.0344,0.0343,0.0312,0.0792,0.0802,5.0715,0f000005,0*2296f550\n\tsystem status\tnormal 2 28.000000 0 0\trobot status\t224.450840\t106.291400\t8.223000\t-0.400588\t-0.588760\t162.076277\t0.000000\t0.000000\n\t\n15:39:52.3\tlog_raw\tgps_raw\t\tsystem status\tnormal 2 28.000000 0 0\trobot status\t224.450995\t106.291133\t8.223000\t-0.402507\t-0.587203\t162.076012\t0.000000\t0.000000\n\t\n15:39:52.8\tlog_raw\tgps_raw\t\tsystem status\tnormal 2 28.000000 0 0\trobot status\t224.451563\t106.291071\t8.222700\t-0.403224\t-0.586327\t162.075953\t0.000000\t0.000000\n\t\n15:39:53.3\tlog_raw\tgps_raw\t#DUALANTENNAHEADINGA,USB3,0,44.5,FINESTEERING,2107,283211.300,02000000,d426,15824;INSUFFICIENT_OBS,NONE,-1.000000000,0.000000000,0.000000000,0.0,0.000000000,0.000000000,\"631T\",14,4,4,3,04,00,20,03*11216130\n\tsystem status\tnormal 2 28.000000 0 0\trobot status\t224.451709\t106.291000\t8.222500\t-0.403685\t-0.587762\t162.075944\t0.000000\t0.000000\n\t\n15:39:53.8\tlog_raw\tgps_raw\t#DUALANTENNAHEADINGA,USB3,0,44.5,FINESTEERING,2107,283211.800,02000000,d426,15824;INSUFFICIENT_OBS,NONE,-1.000000000,0.000000000,0.000000000,0.0,0.000000000,0.000000000,\"631T\",17,4,4,3,04,00,20,03*2745c5ad\n\tsystem status\tnormal 2 28.000000 0 0\trobot status\t224.451496\t106.291494\t8.222300\t-0.402212\t-0.585601\t162.077028\t0.000000\t0.000000\n\t\n15:39:54.3\tlog_raw\tgps_raw\t\tsystem status\tnormal 2 28.000000 0 0\trobot status\t224.451344\t106.291726\t8.222300\t-0.400821\t-0.585524\t162.077872\t0.000000\t0.000000\n\t\n15:39:54.8\tlog_raw\tgps_raw\t#DUALANTENNAHEADINGA,USB3,0,48.0,FINESTEERING,2107,283212.800,02000000,d426,15824;INSUFFICIENT_OBS,NONE,-1.000000000,0.000000000,0.000000000,0.0,0.000000000,0.000000000,\"631T\",17,4,4,3,04,00,20,03*1af1cb79\n\tsystem status\tnormal 2 28.000000 0 0\trobot status\t224.451306\t106.291899\t8.222500\t-0.400151\t-0.584587\t162.076750\t0.000000\t0.000000\n\t\n15:39:55.3\tlog_raw\tgps_raw\t#DUALANTENNAHEADINGA,USB3,0,47.5,FINESTEERING,2107,283213.300,02000000,d426,15824;INSUFFICIENT_OBS,NONE,-1.000000000,0.000000000,0.000000000,0.0,0.000000000,0.000000000,\"631T\",17,4,4,3,04,00,20,03*c50a95c7\n\tsystem status\tnormal 2 28.000000 0 0\trobot status\t224.451384\t106.291635\t8.222800\t-0.398385\t-0.585053\t162.076585\t0.000000\t0.000000\n\t\n15:39:55.8\tlog_raw\tgps_raw\t#INSPVAXA,USB3,0,47.5,FINESTEERING,2107,283213.850,02000000,471d,15824;INS_ALIGNMENT_COMPLETE,INS_RTKFIXED,37.37108793573,126.72336903807,8.2229,22.3000,0.0072,0.0033,-0.0007,-0.395561271,-0.586256352,287.924343856,0.2123,0.1575,0.2642,0.0344,0.0343,0.0312,0.0792,0.0802,5.0774,0f000005,0*129510f9\n\tsystem status\tnormal 2 28.000000 0 0\trobot status\t224.451609\t106.291304\t8.222900\t-0.396055\t-0.585651\t162.076234\t0.000000\t0.000000\n\t\n15:39:56.3\tlog_raw\tgps_raw\t#INSPVAXA,USB3,0,49.0,FINESTEERING,2107,283214.350,02000000,471d,15824;INS_ALIGNMENT_COMPLETE,INS_RTKFIXED,37.37108793342,126.72336903992,8.2230,22.3000,0.0065,0.0039,-0.0008,-0.396825161,-0.583976103,287.925419134,0.2123,0.1575,0.2641,0.0344,0.0343,0.0312,0.0792,0.0802,5.0789,0f000005,0*b5398675\n\tsystem status\tnormal 2 28.000000 0 0\trobot status\t224.451796\t106.291036\t8.223000\t-0.396825\t-0.583976\t162.074581\t0.000000\t0.000000\n\t\n15:39:56.8\tlog_raw\tgps_raw\t#DUALANTENNAHEADINGA,USB3,0,49.0,FINESTEERING,2107,283214.800,02000000,d426,15824;INSUFFICIENT_OBS,NONE,-1.000000000,0.000000000,0.000000000,0.0,0.000000000,0.000000000,\"631T\",14,4,4,3,04,00,20,03*6a4287e3\n\tsystem status\tnormal 2 28.000000 0 0\trobot status\t224.452239\t106.290879\t8.223200\t-0.395713\t-0.583648\t162.076258\t0.000000\t0.000000\n\t\n15:39:57.3\tlog_raw\tgps_raw\t#DUALANTENNAHEADINGA,USB3,0,48.5,FINESTEERING,2107,283215.300,02000000,d426,15824;INSUFFICIENT_OBS,NONE,-1.000000000,0.000000000,0.000000000,0.0,0.000000000,0.000000000,\"631T\",17,4,4,3,04,00,20,03*00c017cf\n\tsystem status\tnormal 2 28.000000 0 0\trobot status\t224.452502\t106.290587\t8.223400\t-0.396465\t-0.585149\t162.076910\t0.000000\t0.000000\n\t\n15:39:57.8\tlog_raw\tgps_raw\t#DUALANTENNAHEADINGA,USB3,0,48.5,FINESTEERING,2107,283215.800,02000000,d426,15824;INSUFFICIENT_OBS,NONE,-1.000000000,0.000000000,0.000000000,0.0,0.000000000,0.000000000,\"631T\",16,4,4,3,04,00,20,03*4210b5a3\n\tsystem status\tnormal 2 28.000000 0 0\trobot status\t224.452907\t106.290429\t8.223700\t-0.396571\t-0.585095\t162.075305\t0.000000\t0.000000\n\t\n15:39:58.3\tlog_raw\tgps_raw\t#DUALANTENNAHEADINGA,USB3,0,44.5,FINESTEERING,2107,283216.300,02000000,d426,15824;INSUFFICIENT_OBS,NONE,-1.000000000,0.000000000,0.000000000,0.0,0.000000000,0.000000000,\"631T\",16,4,4,3,04,00,20,03*bfec7f8f\n\tsystem status\tnormal 2 28.000000 0 0\trobot status\t224.453100\t106.290216\t8.223800\t-0.396326\t-0.584334\t162.073720\t0.000000\t0.000000\n\t\n15:39:58.8\tlog_raw\tgps_raw\t\tsystem status\tnormal 2 28.000000 0 0\trobot status\t224.453242\t106.290060\t8.223900\t-0.395197\t-0.584168\t162.071623\t0.000000\t0.000000\n\t\n15:39:59.3\tlog_raw\tgps_raw\t#DUALANTENNAHEADINGA,USB3,0,49.5,FINESTEERING,2107,283217.300,02000000,d426,15824;INSUFFICIENT_OBS,NONE,-1.000000000,0.000000000,0.000000000,0.0,0.000000000,0.000000000,\"631T\",16,4,4,3,04,00,20,03*68d64881\n\tsystem status\tnormal 2 28.000000 0 0\trobot status\t224.453422\t106.289751\t8.223900\t-0.395984\t-0.584147\t162.071682\t0.000000\t0.000000\n\t\n15:39:59.8\tlog_raw\tgps_raw\t#INSPVAXA,USB3,0,49.5,FINESTEERING,2107,283217.850,02000000,471d,15824;INS_ALIGNMENT_COMPLETE,INS_RTKFIXED,37.37108791854,126.72336906586,8.2236,22.3000,0.0038,0.0069,-0.0005,-0.397358519,-0.581659593,287.929077774,0.2122,0.1575,0.2640,0.0344,0.0343,0.0312,0.0792,0.0802,5.0831,0f000005,0*bf1b0ee9\n\tsystem status\t
